vi "Fast Create Mask By Alpha.vi"(11 "image data":T1) -> (3 "masked image data":T1)   [LabVIEW 2020, in "G-Image.lvlib"]
uses:
  G-Image.lvlib
  <vilib>/picture/picture.llb/imagedata.ctl
panel:
  out "mask":u8[](array[numeric])
  out "*(type *) &x":u8[](array[numeric])
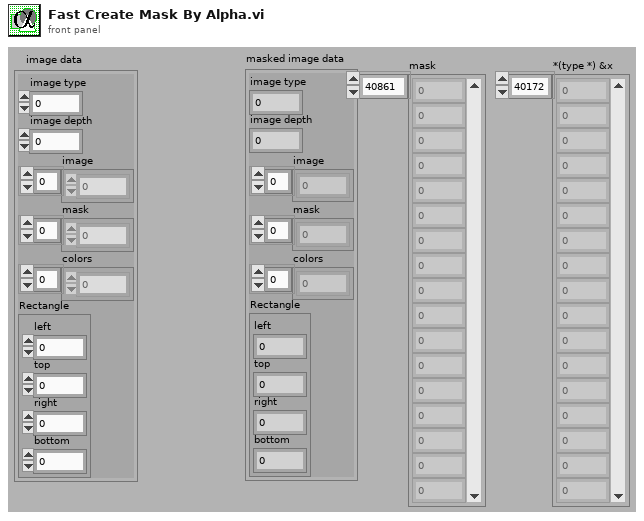
[diagram p1: front panel]
types:
  T1 = typedef "imagedata.ctl" = cluster{"image type":i32, "image depth":i32, "image":u8[], "mask":u8[], "colors":u32[], "Rectangle":cluster{"left":i16, "top":i16, "right":i16, "bottom":i16}}
  T2 = cluster{"left":i16, "top":i16, "right":i16, "bottom":i16}
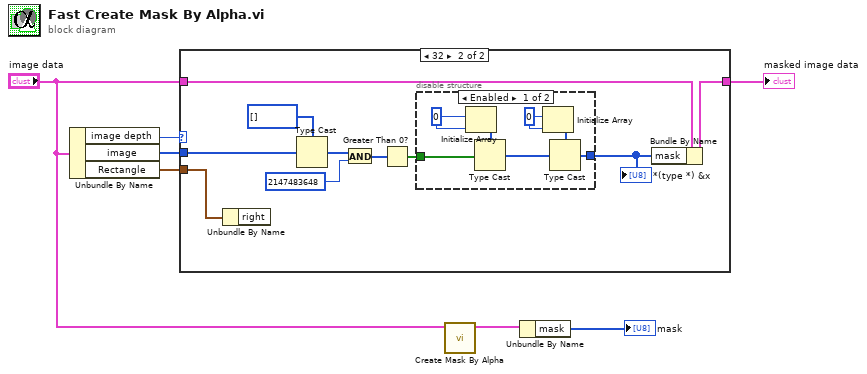
[diagram p0: block diagram]
diagram:
  n1 = Unbundle By Name("image data") -> ("image depth"=w7:i32, "image"=w6:u8[], "Rectangle"=w1:T2)
  n2 = case shown="32" w7 {
    tunnel: w6 -> [_ w16]
    tunnel: "image data" -> [w8 w18]
    tunnel: [w8 w17] -> w5
    tunnel: w1 -> [_ w9]
    frame Default {
    }
    frame 32 {
      n3 = Unbundle By Name(w9) -> ()  [unwired: 1 out]
      n4 = Type Cast(type=u32[] [], x=w16) -> (*(type *) &x=w14:u32[])
      n5 = And(x=w14, y=u32 2147483648) -> (x .and. y?=w12:u32[])
      n6 = Greater Than 0?(x=w12) -> (x > 0?=w11:bool[])
      n7 = disable-structure shown="Enabled" {
        disable-tunnel: w11 -> [w25 _]
        disable-tunnel: [w19 _] -> w10
        frame Enabled {
          w21 = u8 0
          w23 = i16 0
          n8 = Initialize Array(w23, w23) -> (w24:i16[])
          n9 = Type Cast(type=w24, x=w25) -> (*(type *) &x=w22:i16[])
          n10 = Initialize Array(w21, w21) -> (w20:u8[])
          n11 = Type Cast(type=w20, x=w22) -> (*(type *) &x=w19:u8[])
        }
        frame Disabled {
        }
      }
      "*(type *) &x" <- w10
      n12 = Bundle By Name(cluster=w18, "mask"=w10) -> (w17:T1)
    }
  }
  "masked image data" <- w5
  n13 = call <vilib>:"Create Mask By Alpha.vi"("image data"="image data") -> ("masked image data"=w3:T1)  [unwired: 10 in]
  n14 = Unbundle By Name(w3) -> ("mask"=→"mask":u8[])
